vi "Get Adjascents.vi"(9 "Column In":i32, 10 "Row In":i32, 11 "Array In":i32[][](array[numeric])) -> (1 "Columns Out":i32[](array[numeric]), 2 "Rows Out":i32[](array[numeric]), 3 "Adjacent Elements":i32[](array[numeric]))   [LabVIEW 2019, in "Day 11.lvlib"]
uses:
  Day 11.lvlib
  Controls/Side.ctl
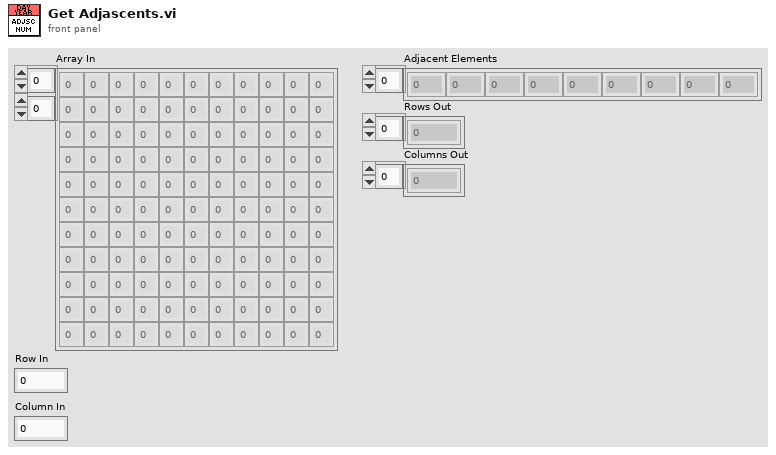
[diagram p1: front panel]
types:
  T1 = typedef "Day 11.lvlib/Side.ctl" = enum16{"Rigth", "Left", "Down", "Up", "Rigth Up", "Rigth Down", "Left Up", "Left Down"}
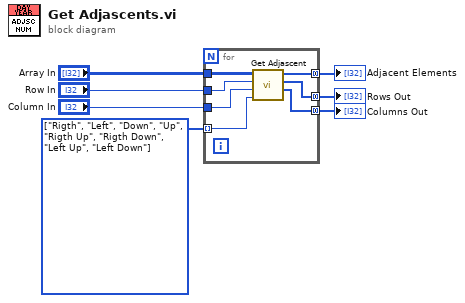
[diagram p0: block diagram]
diagram:
  w3 = T1[] [enum."Rigth", enum."Left", enum."Down", enum."Up", enum."Rigth Up", enum."Rigth Down", enum."Left Up", enum."Left Down"] items=["Rigth", "Left", "Down", "Up", "Rigth Up", "Rigth Down", "Left Up", "Left Down"]
  n1 = for {
    tunnel: "Array In" -> [w14]
    tunnel: "Row In" -> [w13]
    tunnel: [w12] -> w5 mode=concatenating
    tunnel: "Column In" -> [w11]
    tunnel: w3 -> [w10] mode=indexing
    tunnel: [w9] -> w2 mode=concatenating
    tunnel: [w8] -> w1 mode=concatenating
    n2 = call "Get Adjascent.vi"("Side"=w10, "Column Out"=w11, "Row In"=w13, "Array In"=w14) -> ("Column Out"=w8:i32[], "Row Out"=w9:i32[], "Array"=w12:i32[])  [unwired: 5 in]
  }
  "Adjacent Elements" <- w5
  "Rows Out" <- w2
  "Columns Out" <- w1
